vi "Encode IR Parameters.vi"(8 "ADD Parameters (in)":string, 9 "Scanner Settings in":T2={"Scan1"=1, "Scan2"=1, "Scan3"=1, "Scan4"=1, "Scan5"=1, "Scan6"=1, "Scan7"=1, "Scan8"=1, "Scan9"=1, "Scan10"=1, "Scan11"=1, "Scan12"=1, "Scan13"=1, "Scan14"=1, "Scan15"=1, "Scan16"=1} {"Scan16" scale=0.0..2.0; "Scan15" scale=0.0..2.0; "Scan14" scale=0.0..2.0; "Scan13" scale=0.0..2.0; "Scan12" scale=0.0..2.0; "Scan11" scale=0.0..2.0; "Scan10" scale=0.0..2.0; "Scan9" scale=0.0..2.0; "Scan8" scale=0.0..2.0; "Scan7" scale=0.0..2.0; "Scan6" scale=0.0..2.0; "Scan5" scale=0.0..2.0; "Scan4" scale=0.0..2.0; "Scan3" min=0 max=2 scale=0.0..2.0; "Scan2" min=0 max=2 scale=0.0..2.0; "Scan1" min=0 max=2 scale=0.0..2.0}, 10 "Internal Scanner Exists?":bool, 11 "IR Test Parameters in":T1={"Voltage (1000)"=1000, "High Limit(0.0, 0.5 - 50000 Megohms) (5)"=0.0, "Low Limit(0.1 - 50000 Megohms) (0)"=0.1, "Ramp Up Time (0.1 - 999.9 seconds) (0.1)"=0.1, "Delay Time (0.0, 1.0 - 999.9 seconds) (0.5)"=0.5, "Ramp Down Time (0.0 - 999.9 seconds) (0) "=0.0, "Charge LO (0)"=0.0, "Auto Charge LO (F: Off)"=FALSE, "Dwell Time (0.0, 1.0 - 999.9 seconds) (0.5)"=0.5} {"Dwell Time (0.0, 1.0 - 999.9 seconds) (0.5)" format="%.1f"; "Ramp Down Time (0.0 - 999.9 seconds) (0)" format="%.1f"; "Charge LO (0)" format="%.2f"; "Delay Time (0.0, 1.0 - 999.9 seconds) (0.5)" format="%.1f"; "Ramp Up Time (0.1 - 999.9 seconds) (0.1)" format="%.1f"; "Low Limit(0.1 - 50000 Megohms) (0)" format="%.1f"; "High Limit(0.0, 0.5 - 50000 Megohms) (5)" format="%.1f"}) -> (1 "Scanner Settings out":T2={"Scan1"=1, "Scan2"=1, "Scan3"=1, "Scan4"=1, "Scan5"=1, "Scan6"=1, "Scan7"=1, "Scan8"=1, "Scan9"=1, "Scan10"=1, "Scan11"=1, "Scan12"=1, "Scan13"=1, "Scan14"=1, "Scan15"=1, "Scan16"=1} {"Scan16" scale=0.0..2.0; "Scan15" scale=0.0..2.0; "Scan14" scale=0.0..2.0; "Scan13" scale=0.0..2.0; "Scan12" scale=0.0..2.0; "Scan11" scale=0.0..2.0; "Scan10" scale=0.0..2.0; "Scan9" scale=0.0..2.0; "Scan8" scale=0.0..2.0; "Scan7" scale=0.0..2.0; "Scan6" scale=0.0..2.0; "Scan5" scale=0.0..2.0; "Scan4" scale=0.0..2.0; "Scan3" min=0 max=2 scale=0.0..2.0; "Scan2" min=0 max=2 scale=0.0..2.0; "Scan1" min=0 max=2 scale=0.0..2.0}, 2 "IR Test Parameters out":T1={"Voltage (1000)"=1000, "High Limit(0.0, 0.5 - 50000 Megohms) (5)"=0.0, "Low Limit(0.1 - 50000 Megohms) (0)"=0.1, "Ramp Up Time (0.1 - 999.9 seconds) (0.1)"=0.1, "Delay Time (0.0, 1.0 - 999.9 seconds) (0.5)"=0.5, "Ramp Down Time (0.0 - 999.9 seconds) (0) "=0.0, "Charge LO (0)"=0.0, "Auto Charge LO (F: Off)"=FALSE, "Dwell Time (0.0, 1.0 - 999.9 seconds) (0.5)"=0.5} {"Dwell Time (0.0, 1.0 - 999.9 seconds) (0.5)" format="%.1f"; "Ramp Down Time (0.0 - 999.9 seconds) (0)" format="%.1f"; "Charge LO (0)" format="%.2f"; "Delay Time (0.0, 1.0 - 999.9 seconds) (0.5)" format="%.1f"; "Ramp Up Time (0.1 - 999.9 seconds) (0.1)" format="%.1f"; "Low Limit(0.1 - 50000 Megohms) (0)" format="%.1f"; "High Limit(0.0, 0.5 - 50000 Megohms) (5)" format="%.1f"}, 3 "ADD command":string)   [LabVIEW 2020, in "Associated Research 78XX Series.lvlib"]
uses:
  <instrlib>/Associated Research 78XX Series/Associated Research 78XX Series.lvlib
  <instrlib>/Associated Research 78XX Series/Public/Configure/Steps/Low Level/Scanner Settings.ctl
  <instrlib>/Associated Research 78XX Series/Public/Configure/Steps/Low Level/IR Test Parameters.ctl
panel:
  # "On\nOff"
  # "On\nOff"
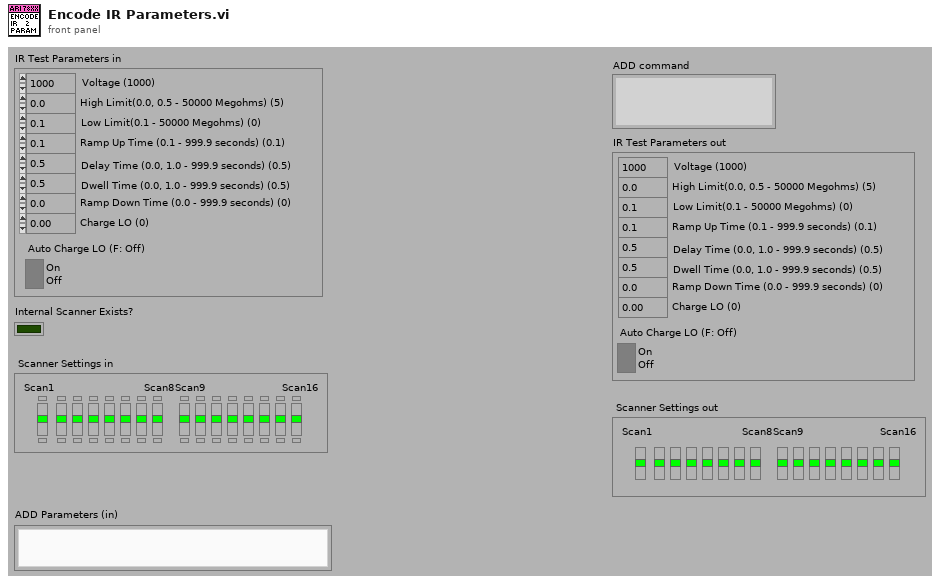
[diagram p1: front panel]
types:
  T1 = typedef "Associated Research 78XX Series.lvlib/IR Test Parameters.ctl" = cluster{"Voltage (1000)":i32, "High Limit(0.0, 0.5 - 50000 Megohms) (5)":dbl, "Low Limit(0.1 - 50000 Megohms) (0)":dbl, "Ramp Up Time (0.1 - 999.9 seconds) (0.1)":dbl, "Delay Time (0.0, 1.0 - 999.9 seconds) (0.5)":dbl, "Ramp Down Time (0.0 - 999.9 seconds) (0) ":dbl, "Charge LO (0)":dbl, "Auto Charge LO (F: Off)":bool, "Dwell Time (0.0, 1.0 - 999.9 seconds) (0.5)":dbl}
  T2 = typedef "Associated Research 78XX Series.lvlib/Scanner Settings.ctl" = cluster{"Scan1":i32, "Scan2":i32, "Scan3":i32, "Scan4":i32, "Scan5":i32, "Scan6":i32, "Scan7":i32, "Scan8":i32, "Scan9":i32, "Scan10":i32, "Scan11":i32, "Scan12":i32, "Scan13":i32, "Scan14":i32, "Scan15":i32, "Scan16":i32}
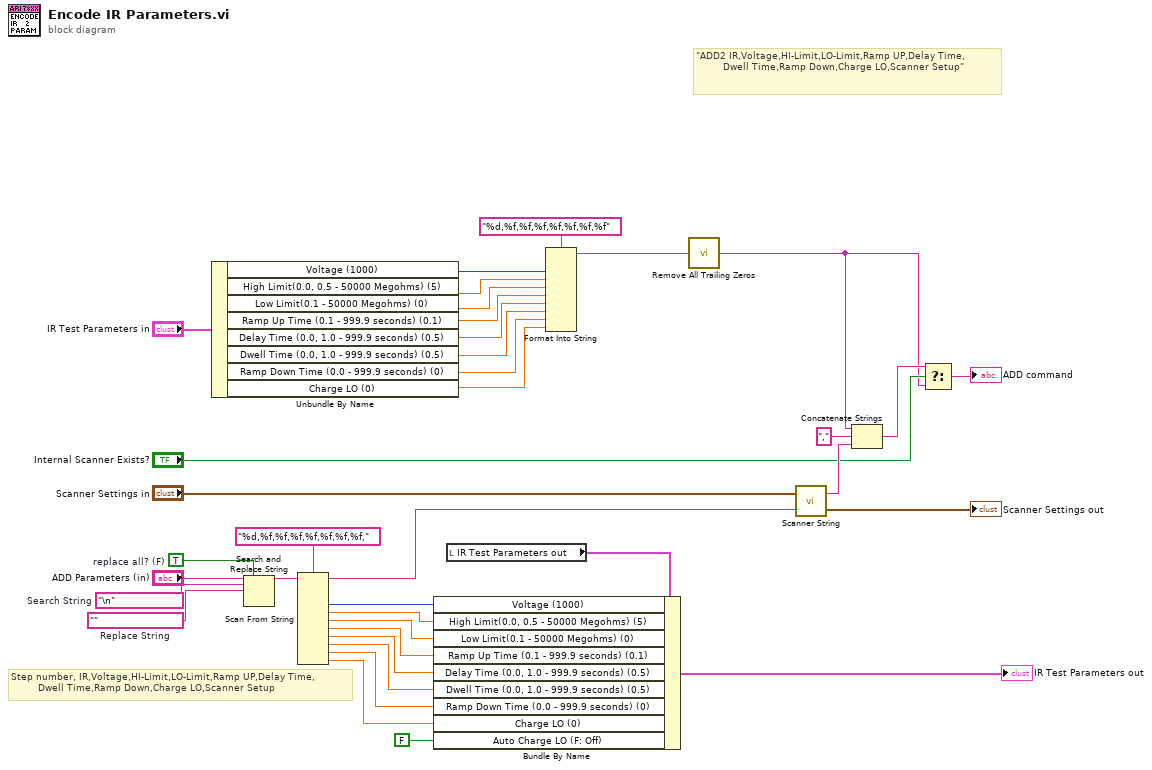
[diagram p0: block diagram]
diagram:
  w15 = TRUE  # replace all? (F)
  w16 = ""  # Replace String
  w17 = "\n"  # Search String
  # "Step number, IR,Voltage,HI-Limit,LO-Limit,Ramp UP,Delay Time,\n         Dwell Time,Ramp Down,Charge LO,Scanner Setup"
  # "\"ADD2 IR,Voltage,HI-Limit,LO-Limit,Ramp UP,Delay Time,\n         Dwell Time,Ramp Down,Charge LO,Scanner Setup\""
  n1 = Unbundle By Name("IR Test Parameters in") -> ("Voltage (1000)"=w37:i32, "High Limit(0.0, 0.5 - 50000 Megohms) (5)"=w36:dbl, "Low Limit(0.1 - 50000 Megohms) (0)"=w35:dbl, "Ramp Up Time (0.1 - 999.9 seconds) (0.1)"=w34:dbl, "Delay Time (0.0, 1.0 - 999.9 seconds) (0.5)"=w10:dbl, "Dwell Time (0.0, 1.0 - 999.9 seconds) (0.5)"=w33:dbl, "Ramp Down Time (0.0 - 999.9 seconds) (0)"=w32:dbl, "Charge LO (0)"=w31:dbl)
  n2 = Search and Replace String(replace all?=w15, input string="ADD Parameters (in)", search string=w17, replace string=w16) -> (result string=w13:string)  [unwired: 4 in, 3 out]
  n3 = Scan From String(format string="%d,%f,%f,%f,%f,%f,%f,%f," ("Format String"), input string=w13) -> (remaining string=w7:string, output 1=w23:i32, output 2=w12:dbl, output 3=w22:dbl, output 4=w21:dbl, output 5=w9:dbl, output 6=w11:dbl, output 7=w20:dbl, output 8=w19:dbl)  [unwired: 10 in, 2 out]
  n4 = local read "IR Test Parameters out"() -> (w2:T1)
  n5 = Bundle By Name(cluster=w2, "Voltage (1000)"=w23, "High Limit(0.0, 0.5 - 50000 Megohms) (5)"=w12, "Low Limit(0.1 - 50000 Megohms) (0)"=w22, "Ramp Up Time (0.1 - 999.9 seconds) (0.1)"=w21, "Delay Time (0.0, 1.0 - 999.9 seconds) (0.5)"=w9, "Dwell Time (0.0, 1.0 - 999.9 seconds) (0.5)"=w11, "Ramp Down Time (0.0 - 999.9 seconds) (0)"=w20, "Charge LO (0)"=w19, "Auto Charge LO (F: Off)"=FALSE) -> (→"IR Test Parameters out":T1)
  n6 = Format Into String(format string="%d,%f,%f,%f,%f,%f,%f,%f" ("Format String"), w37, w36, w35, w34, w10, w33, w32, w31) -> (resulting string=w27:string)  [unwired: 2 in, 1 out]
  n7 = call <instrlib>:"Remove All Trailing Zeros.vi"("String in"=w27) -> ("String out"=w8:string)
  n8 = call <instrlib>:"Scanner String.vi"("Scanner String (in)"=w7, "Scanner Settings in"="Scanner Settings in") -> ("Scanner Settings out"=→"Scanner Settings out":T2, "Scanner String (out)"=w29:string)
  n9 = Concatenate Strings(w8, "," ("Substring"), w29) -> (w25:string)
  n10 = Select(t=w25, s="Internal Scanner Exists?", f=w8) -> (s? t:f=→"ADD command":string)
